vi "Second Call.vi"() -> (0 "Second Call?: T/F":bool)   [LabVIEW 2017]
doc: "Returns TRUE only on the second call after the Run button is clicked, and FALSE on every other call."
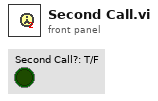
[diagram p1: front panel]
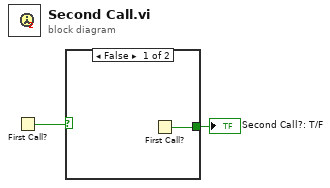
[diagram p0: block diagram]
diagram:
  n1 = First Call?() -> (First Call?: T/F=w2:bool)
  n2 = case shown="False" w2 {
    tunnel: [w3 _] -> w1
    frame False {
      n3 = First Call?() -> (First Call?: T/F=w3:bool)
    }
    frame True {
    }
  }
  "Second Call?: T/F" <- w1
